vi "HXG2_PowerUncert.vi"(0 "Tout Liq (°F)":dbl, 1 "Cp (BTU/lbm °F)":dbl, 2 "Mass Flow (lbm/hr)":dbl, 3 "Inlet Temp Uncert (°F)":dbl=0.09, 4 "Outlet Temp Uncert (°F)":dbl=0.09, 5 "error in (no error)":errorcluster, 6 "Tin Liq (°F)":dbl, 7 "% of rate specs":dbl[](array[numeric])) -> (14 "Uncertainty Calcs":T1 {"% error T" format="%#.3f"; "% error Power" format="%#.3f"; "% error Mdot" format="%#.3f"; "Power Uncert (BTU/hr)" format="%#.3f"; "Power Uncert (W)" format="%#.3f"}, 19 "error out":errorcluster)   [LabVIEW 2012]
panel:
  out "Power Uncert (W)":dbl format="%#.3f"
  out "% error Power":dbl format="%#.3f"
  out "Power Uncert (BTU/hr)":dbl format="%#.3f"
  out "Power (BTU/hr)":dbl
  out "% error T":dbl format="%#.3f"
  out "% error Mdot":dbl format="%#.3f"
  out "Mass Flow Uncert (lbm/hr)":dbl format="%#.3f"
  # "MicroMotion ELITE mass flow meters:"
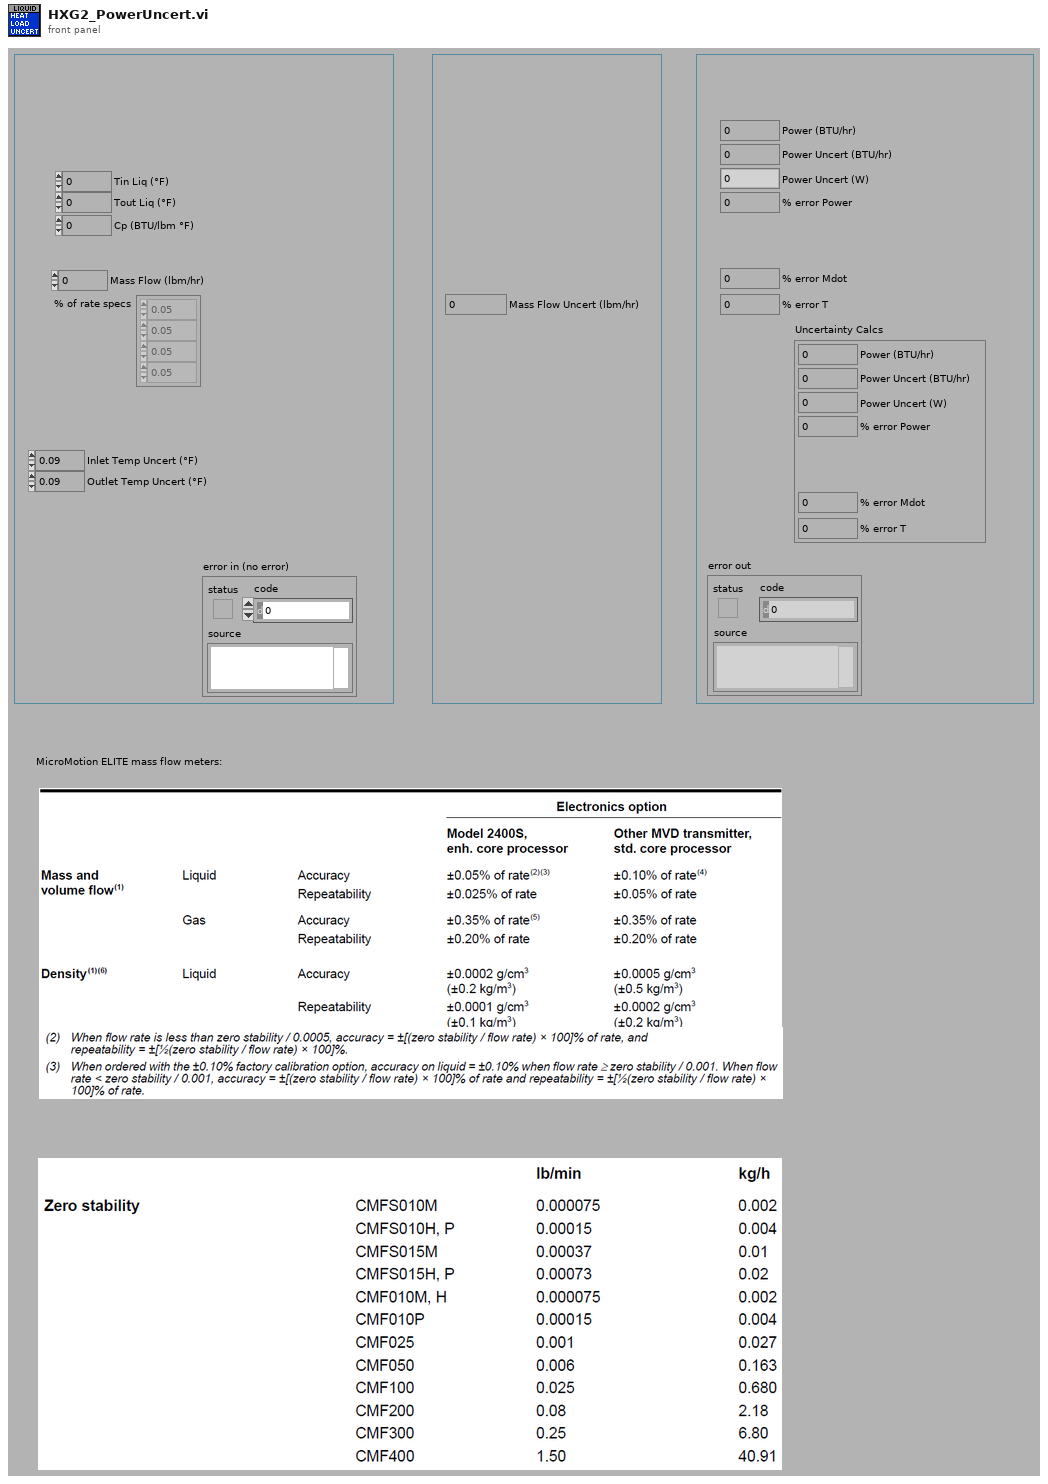
[diagram p1: front panel]
types:
  T1 = cluster{"Power (BTU/hr)":dbl, "Power Uncert (W)":dbl, "Power Uncert (BTU/hr)":dbl, "% error Mdot":dbl, "% error Power":dbl, "% error T":dbl}
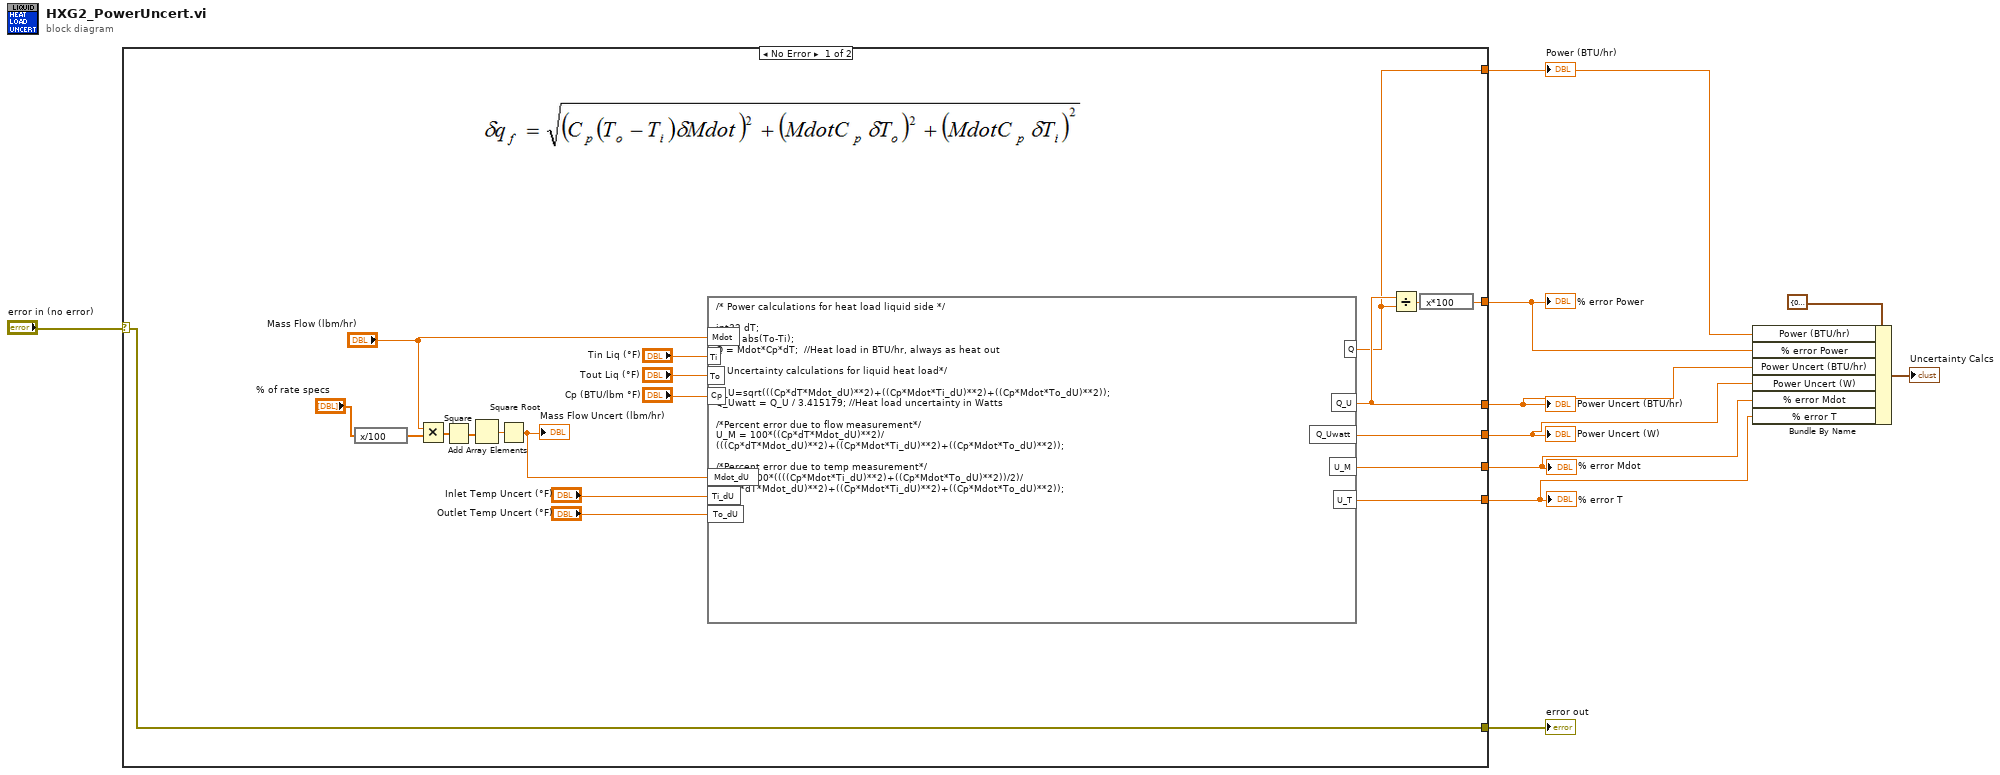
[diagram p0: block diagram]
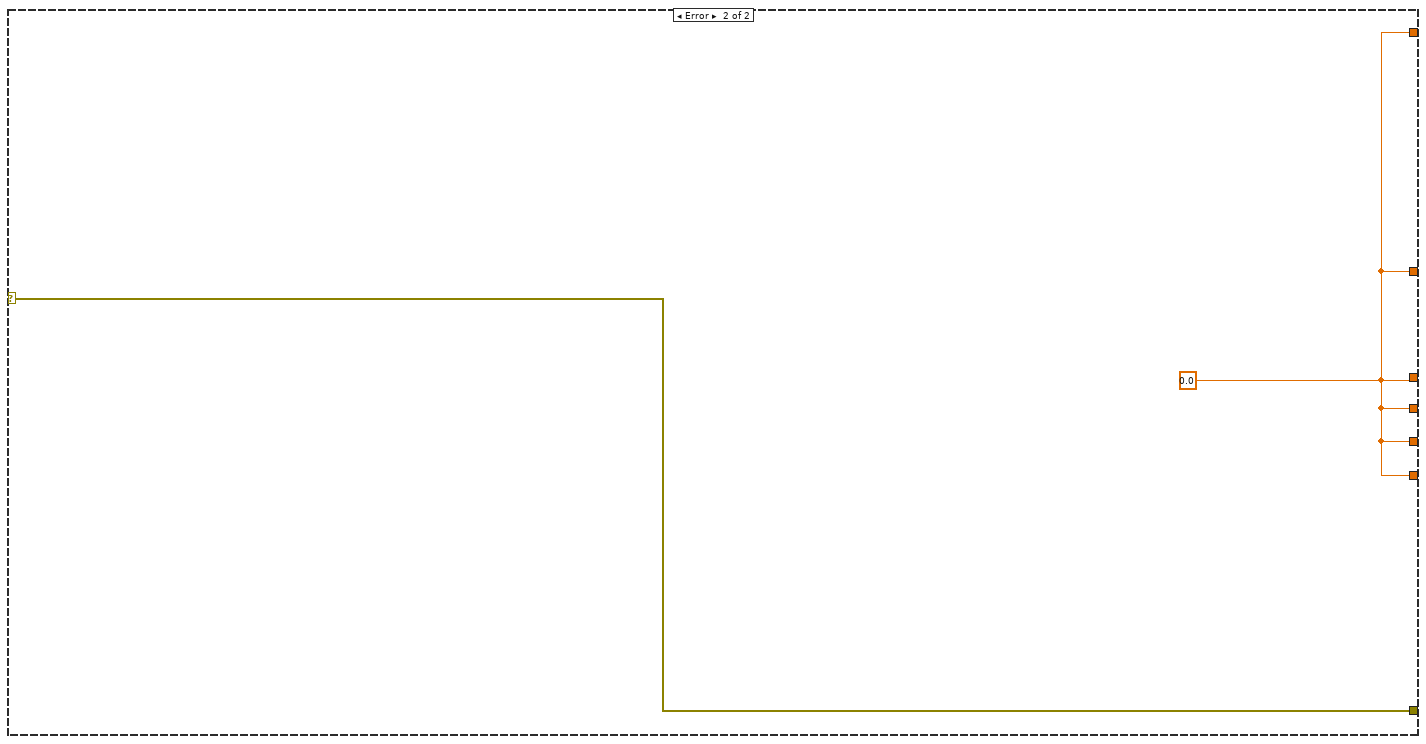
[diagram p2: hidden frame]
diagram:
  n1 = case shown="No Error" "error in (no error)" {
    selector: "error in (no error)" -> [w30 w32]
    tunnel: [w30 w32] -> w10
    tunnel: [w16 w31] -> w4
    tunnel: [w29 w31] -> w3
    tunnel: [w13 w31] -> w5
    tunnel: [w14 w31] -> w6
    tunnel: [w12 w31] -> w1
    tunnel: [w11 w31] -> w2
    frame No Error {
      n2 = expression code="x/100"("% of rate specs") -> (w19:dbl[])
      n3 = Multiply(x="Mass Flow (lbm/hr)", y=w19) -> (x*y=w21:dbl[])
      n4 = Square(x=w21) -> (x^2=w23:dbl[])
      n5 = Add Array Elements(numeric array=w23) -> (sum=w22:dbl)
      n6 = Square Root(x=w22) -> (sqrt(x)=w18:dbl)
      "Mass Flow Uncert (lbm/hr)" <- w18
      n7 = formula code="/* Power calculations for heat load liquid side */\n\nint32 dT;\ndT = abs(To-Ti); \nQ = Mdot*Cp*dT;  //Heat load in BTU/hr, always as heat out\n\n/* Uncertainty calculations for liquid heat load*/\n\nQ_U=sqrt(((Cp*dT*Mdot_dU)**2)+((Cp*Mdot*Ti_dU)**2)+((Cp*Mdot*To_dU)**2));\nQ_Uwatt = Q_U / 3.415179; //Heat load uncertainty in Watts\n\n/*Percent error due to flow measurement*/\nU_M = 100*((Cp*dT*Mdot_dU)**2)/\n(((Cp*dT*Mdot_dU)**2)+((Cp*Mdot*Ti_dU)**2)+((Cp*Mdot*To_dU)**2));\n\n/*Percent error due to temp measurement*/\nU_T =  100*((((Cp*Mdot*Ti_dU)**2)+((Cp*Mdot*To_dU)**2))/2)/\n(((Cp*dT*Mdot_dU)**2)+((Cp*Mdot*Ti_dU)**2)+((Cp*Mdot*To_dU)**2));"("Mdot"="Mass Flow (lbm/hr)", "Ti"="Tin Liq (°F)", "To"="Tout Liq (°F)", "Cp"="Cp (BTU/lbm °F)", "Ti_dU"="Inlet Temp Uncert (°F)", "To_dU"="Outlet Temp Uncert (°F)", "Mdot_dU"=w18) -> ("Q_U"=w16:dbl, "Q_Uwatt"=w29:dbl, "Q"=w14:dbl, "U_M"=w11:dbl, "U_T"=w12:dbl)
      n8 = Divide(x=w16, y=w14) -> (x/y=w15:dbl)
      n9 = expression code="x*100"(w15) -> (w13:dbl)
    }
    frame Error {
      w31 = 0.0 ("Q_U")
    }
  }
  "error out" <- w10
  "% error T" <- w1
  "% error Power" <- w5
  "% error Mdot" <- w2
  "Power Uncert (BTU/hr)" <- w4
  "Power Uncert (W)" <- w3
  "Power (BTU/hr)" <- w6
  n10 = Bundle By Name(cluster=T1 {"Power (BTU/hr)"=0.0, "Power Uncert (W)"=0.0, "Power Uncert (BTU/hr)"=0.0, "% error Mdot"=0.0, "% error Power"=0.0, "% error T"=0.0} ("Uncertainty Calcs"), "Power (BTU/hr)"=w6, "% error Power"=w5, "Power Uncert (BTU/hr)"=w4, "Power Uncert (W)"=w3, "% error Mdot"=w2, "% error T"=w1) -> (→"Uncertainty Calcs":T1)
